vi "输入数据解析.vi"(0 "单个参数补充":dbl, 1 "从板号":dbl=1.0, 2 "主板二维码":string="BNET01", 3 "从板二维码":string="BNET01", 5 "主板引用":refnum<vi>, 7 "从板引用":refnum<vi>, 9 "主板选项":string="三级故障阀值", 11 "枚举":enum16{"主板", "从板"}(ring), 12 "快换":bool caption="快换写入") -> (4 "输出数组":dbl[][](array[numeric]), 6 "数组长度":dbl[](array[numeric]), 8 "循环次数":i32, 10 "命令":u32, 14 "名称":string[](array[string]), 15 "命令序号":u32[](array[numeric]))   [LabVIEW 2013] (continued)
          n307 = Build Array(u32 5 ("命令序号")) -> (w669:u32[])
          n308 = Insert Into Array(array=w655, index=w657, new element #1=w657, new element #2=1.0 ("新元素/子数组")) -> (w656:dbl[])
          n309 = Build Array(w656) -> (w664:dbl[][])
          n310 = Build Array("温度个数") -> (w660:string[])
        }
        frame "温度起始值" {
          n311 = Unbundle By Name(w709) -> ("项目信息"=w704:refnum<vi>)
          n312 = property class="Tbl (严格)"(reference=w704) -> ("Value"=w703:string[][])  [unwired: 1 in, 2 out]
          n313 = Index Array(array=w703, index (col)=1 ("禁用的索引 (列)")) -> (element=w705:string[])  [unwired: 1 in]
          n314 = Increment(x=w696) -> (x+1=w698:dbl)
          n315 = Multiply(x=w696, y=3.0) -> (x*y=w694:dbl)
          n316 = Add(x=w694, y=23.0) -> (x+y=w697:dbl)
          n317 = Array Subset(array=w705, index=w697, length=w698) -> (w707:string[])
          n318 = Fract/Exp String To Number(string=w707) -> (number=w692:dbl[])  [unwired: 4 out]
          n319 = for {
            tunnel: w692 -> [w716] mode=indexing
            shift-right: [w711] -> w691
            shift-left: dbl[] [] -> [w710]
            n320 = Quotient & Remainder(x=w716, y=256.0) -> (x-y*floor(x/y)=w713:dbl, floor(x/y)=w714:dbl)
            n321 = Build Array(w714, w713) -> (w712:dbl[])
            n322 = Insert Into Array(array=w710, new element=w712) -> (w711:dbl[])  [unwired: 1 in]
          }
          n323 = Build Array(62.0 ("元素")) -> (w702:dbl[])
          n324 = Build Array(u32 6 ("命令序号")) -> (w700:u32[])
          n325 = Build Array(w691) -> (w690:dbl[][])
          n326 = Build Array("温度起始值") -> (w686:string[])
        }
        frame "SOC" {
          # "SOC"
          n327 = Unbundle By Name(w737) -> ("一级故障 4"=w732:refnum<vi>)
          n328 = property class="Clust (严格)"(reference=w732) -> ("Value"=w731:T3)  [unwired: 1 in, 2 out]
          n329 = Unbundle By Name(w731) -> ("SOC(%)"=w729:dbl)
          n330 = call "输入分辨率计算-EV05.vi"("1字节?"=FALSE, "数值"=w729, "分辨率"=0.1) -> ("低字节"=w726:dbl, "高字节1"=w727:dbl)  [unwired: 2 in, 5 out]
          n331 = Build Array(w727, w726) -> (w738:dbl[])
          n332 = Two Button Dialog(message="输入SOC前请确认实际容量己输入" ("消息"), 1:"取消" ("F按钮名称（“取消”）"), 2:"确定" ("T按钮名称（“确定”）")) -> (T button?=w720:bool)
          n333 = case shown="假" w720 {
            tunnel: [0 1] -> w733
            frame False {
            }
            frame True {
            }
          }
          n334 = Build Array("SOC") -> (w721:string[])
          n335 = Build Array(w738) -> (w725:dbl[][])
          n336 = Build Array(2.0 ("单个参数补充")) -> (w724:dbl[])
          n337 = Build Array(u32 7 ("命令序号")) -> (w723:u32[])
        }
        frame "电池额定实际容量" {
          w754 = 256.0 ("y")
          w763 = 256.0 ("y")
          # "电池额定容量,实际容量"
          n338 = Unbundle By Name(w774) -> ("一级故障 4"=w761:refnum<vi>)
          n339 = property class="Clust (严格)"(reference=w761) -> ("Value"=w760:T3)  [unwired: 1 in, 2 out]
          n340 = Unbundle By Name(w760) -> ("电池额定容量(A)"=w758:dbl, "电池实际容量(A)"=w757:dbl)
          n341 = call "输入分辨率计算-EV05.vi"("1字节?"=TRUE, "数值 2"=w757, "数值"=w758, "分辨率"=0.001) -> ("高字节 2"=w750:dbl, "高字节1"=w756:dbl)  [unwired: 1 in, 5 out]
          n342 = Quotient & Remainder(x=w756, y=w763) -> (x-y*floor(x/y)=w767:dbl, floor(x/y)=w769:dbl)
          n343 = Quotient & Remainder(x=w750, y=w754) -> (x-y*floor(x/y)=w746:dbl, floor(x/y)=w751:dbl)
          n344 = Quotient & Remainder(x=w769, y=w763) -> (x-y*floor(x/y)=w766:dbl, floor(x/y)=w768:dbl)
          n345 = Quotient & Remainder(x=w751, y=w754) -> (x-y*floor(x/y)=w747:dbl, floor(x/y)=w752:dbl)
          n346 = Quotient & Remainder(x=w768, y=w763) -> (x-y*floor(x/y)=w765:dbl, floor(x/y)=w764:dbl)
          n347 = Quotient & Remainder(x=w752, y=w754) -> (x-y*floor(x/y)=w748:dbl, floor(x/y)=w753:dbl)
          n348 = Quotient & Remainder(x=w753, y=w754) -> (x-y*floor(x/y)=w749:dbl)  [unwired: 1 out]
          n349 = Quotient & Remainder(x=w764, y=w763) -> (x-y*floor(x/y)=w762:dbl)  [unwired: 1 out]
          n350 = Build Array(w762, w765, w766, w767, w749, w748, w747, w746) -> (w775:dbl[])
          n351 = Build Array(w775) -> (w745:dbl[][])
          n352 = Build Array(8.0 ("单个参数补充")) -> (w744:dbl[])
          n353 = Build Array(u32 8 ("命令序号")) -> (w743:u32[])
          n354 = Build Array("电池额定实际容量") -> (w741:string[])
        }
        frame "配置文件版本" {
          w787 = 8 ("长度")
          # "配置文件版本"
          n355 = Unbundle By Name(w789) -> ("一级故障 4"=w783:refnum<vi>)
          n356 = property class="Clust (严格)"(reference=w783) -> ("Value"=w782:T3)  [unwired: 1 in, 2 out]
          n357 = Unbundle By Name(w782) -> ("配置文件版本"=w781:string)
          n358 = String To Byte Array(string=w781) -> (unsigned byte array=w784:u8[])
          n359 = Array Subset(array=w784, length=w787) -> (w790:u8[])  [unwired: 1 in]
          n360 = Build Array(w790) -> (w780:u8[][])
          n361 = Build Array(w787) -> (w779:i32[])
          n362 = Build Array(u32 9 ("命令序号")) -> (w778:u32[])
          n363 = Build Array("配置文件版本") -> (w776:string[])
        }
        frame "参数修改记录" {
          n364 = Unbundle By Name(w813) -> ("一级故障 4"=w802:refnum<vi>)
          n365 = property class="Clust (严格)"(reference=w802) -> ("Value"=w801:T3)  [unwired: 1 in, 2 out]
          n366 = Unbundle By Name(w801) -> ("使用者"=w800:dbl)
          n367 = Quotient & Remainder(x=w800, y=256.0) -> (x-y*floor(x/y)=w797:dbl, floor(x/y)=w798:dbl)
          n368 = call "当前时间解析-8.6.vi"("需要秒？(T)"=TRUE) -> ("年"=w808:u8, "月"=w807:u8, "日"=w806:u8, "时"=w805:u8, "分"=w804:u8, "秒"=w803:u8)  [unwired: 13 out]
          n369 = Build Array(w798, w797, w808, w807, w806, w805, w804, w803) -> (w814:dbl[])
          n370 = Build Array(w814) -> (w796:dbl[][])
          n371 = Build Array(8.0 ("单个参数补充")) -> (w795:dbl[])
          n372 = Build Array(u32 10 ("命令序号")) -> (w794:u32[])
          n373 = Build Array("参数修改记录") -> (w791:string[])
        }
        frame "校正时钟" {
          n374 = call "当前时间解析-8.6.vi"("需要秒？(T)"=TRUE) -> ("年"=w826:u8, "月"=w825:u8, "日"=w824:u8, "时"=w823:u8, "分"=w822:u8, "秒"=w821:u8)  [unwired: 13 out]
          n375 = Build Array(w826, w825, w824, w823, w822, w821) -> (w831:u8[])
          n376 = Build Array(w831) -> (w820:u8[][])
          n377 = Build Array(6.0 ("单个参数补充")) -> (w819:dbl[])
          n378 = Build Array(u32 14 ("命令序号")) -> (w818:u32[])
          n379 = Build Array("校正时钟") -> (w815:string[])
        }
        frame "车牌号" {
          w843 = 8 ("长度")
          # "车牌号"
          n380 = Unbundle By Name(w845) -> ("一级故障 4"=w839:refnum<vi>)
          n381 = property class="Clust (严格)"(reference=w839) -> ("Value"=w838:T3)  [unwired: 1 in, 2 out]
          n382 = Unbundle By Name(w838) -> ("车架(牌)号"=w837:string)
          n383 = String To Byte Array(string=w837) -> (unsigned byte array=w840:u8[])
          n384 = Array Subset(array=w840, length=w843) -> (w846:u8[])  [unwired: 1 in]
          n385 = Build Array(w846) -> (w836:u8[][])
          n386 = Build Array(w843) -> (w835:i32[])
          n387 = Build Array("车牌号") -> (w832:string[])
          n388 = Build Array(u32 11 ("命令序号")) -> (w834:u32[])
        }
        frame "SOH" {
          n389 = Unbundle By Name(w863) -> ("一级故障 4"=w858:refnum<vi>)
          n390 = property class="Clust (严格)"(reference=w858) -> ("Value"=w857:T3)  [unwired: 1 in, 2 out]
          n391 = Unbundle By Name(w857) -> ("SOH(%)"=w856:dbl)
          n392 = call "输入分辨率计算-EV05.vi"("1字节?"=FALSE, "数值"=w856, "分辨率"=0.1) -> ("低字节"=w852:dbl, "高字节1"=w853:dbl)  [unwired: 2 in, 5 out]
          n393 = Build Array(w853, w852) -> (w864:dbl[])
          n394 = Build Array(w864) -> (w851:dbl[][])
          n395 = Build Array(2.0 ("单个参数补充")) -> (w850:dbl[])
          n396 = Build Array("SOH") -> (w847:string[])
          n397 = Build Array(u32 12 ("命令序号")) -> (w849:u32[])
        }
        frame "一级故障阀值" {
          n398 = Unbundle By Name(w870) -> ("一级故障"=w871:refnum<vi>)
          n399 = property class="Clust (严格)"(reference=w871) -> ("Value"=w869:T4)  [unwired: 1 in, 2 out]
          n400 = for {
            N: 17 -> [_]
            tunnel: w869 -> [w881]
            shift-right: [w878] -> w875
            shift-left: dbl[] [] -> [w879]
            i -> [w882]
            n401 = case shown="11" w882 {
              tunnel: w881 -> [w884 w891 w898 w905 w912 w918 w926 w934 w942 w950 w958 w966 w974 w982 w992 w999 w1003]
              tunnel: [w885 w892 w900 w907 w913 w921 w929 w937 w945 w953 w961 w967 w976 w984 w991 w998 w1005] -> w880
              frame 0, Default {
                # "总电压过高"
                n402 = Unbundle By Name(w884) -> ("总电压过高"=w883:dbl)
                n403 = call "输入分辨率计算-EV05.vi"("1字节?"=FALSE, "数值"=w883, "分辨率"=0.1) -> ("低字节"=w887:dbl, "高字节1"=w886:dbl)  [unwired: 2 in, 5 out]
                n404 = Build Array(w886, w887) -> (w885:dbl[])
              }
              frame 1 {
                # "总电压过低"
                n405 = Unbundle By Name(w891) -> ("总电压过低"=w890:dbl)
                n406 = call "输入分辨率计算-EV05.vi"("1字节?"=FALSE, "数值"=w890, "分辨率"=0.1) -> ("低字节"=w894:dbl, "高字节1"=w893:dbl)  [unwired: 2 in, 5 out]
                n407 = Build Array(w893, w894) -> (w892:dbl[])
              }
              frame 2 {
                # "温度过高"
                n408 = Unbundle By Name(w898) -> ("温度过高"=w897:dbl)
                n409 = call "输入分辨率计算-EV05.vi"("1字节?"=TRUE, "数值"=w897, "偏移量"=-40.0, "分辨率"=1.0) -> ("高字节1"=w901:dbl)  [unwired: 1 in, 6 out]
                n410 = Build Array(w901) -> (w900:dbl[])
              }
              frame 3 {
                # "温度过低"
                n411 = Unbundle By Name(w905) -> ("温度过低"=w904:dbl)
                n412 = call "输入分辨率计算-EV05.vi"("1字节?"=TRUE, "数值"=w904, "偏移量"=-40.0, "分辨率"=1.0) -> ("高字节1"=w908:dbl)  [unwired: 1 in, 6 out]
                n413 = Build Array(w908) -> (w907:dbl[])
              }
              frame 4 {
                # "整组温度不均衡"
                n414 = Unbundle By Name(w912) -> ("整组温度不均衡"=w911:dbl)
                n415 = call "输入分辨率计算-EV05.vi"("1字节?"=TRUE, "数值"=w911, "分辨率"=1.0) -> ("高字节1"=w914:dbl)  [unwired: 2 in, 6 out]
                n416 = Build Array(w914) -> (w913:dbl[])
              }
              frame 5 {
                # "单组电压不均衡"
                n417 = Unbundle By Name(w918) -> ("单组电压不均衡"=w917:dbl)
                n418 = call "输入分辨率计算-EV05.vi"("1字节?"=FALSE, "数值"=w917, "偏移量"=0.0, "分辨率"=0.001) -> ("低字节"=w919:dbl, "高字节1"=w922:dbl)  [unwired: 1 in, 5 out]
                n419 = Build Array(w922, w919) -> (w921:dbl[])
              }
              frame 6 {
                # "整组电压不均衡"
                n420 = Unbundle By Name(w926) -> ("整组电压不均衡"=w925:dbl)
                n421 = call "输入分辨率计算-EV05.vi"("1字节?"=FALSE, "数值"=w925, "偏移量"=0.0, "分辨率"=0.001) -> ("低字节"=w927:dbl, "高字节1"=w930:dbl)  [unwired: 1 in, 5 out]
                n422 = Build Array(w930, w927) -> (w929:dbl[])
              }
              frame 7 {
                # "单体电压过高"
                n423 = Unbundle By Name(w934) -> ("单体电压过高"=w933:dbl)
                n424 = call "输入分辨率计算-EV05.vi"("1字节?"=FALSE, "数值"=w933, "偏移量"=0.0, "分辨率"=0.001) -> ("低字节"=w935:dbl, "高字节1"=w938:dbl)  [unwired: 1 in, 5 out]
                n425 = Build Array(w938, w935) -> (w937:dbl[])
              }
              frame 8 {
                # "单体电压过低"
                n426 = Unbundle By Name(w942) -> ("单体电压过低"=w941:dbl)
                n427 = call "输入分辨率计算-EV05.vi"("1字节?"=FALSE, "数值"=w941, "偏移量"=0.0, "分辨率"=0.001) -> ("低字节"=w943:dbl, "高字节1"=w946:dbl)  [unwired: 1 in, 5 out]
                n428 = Build Array(w946, w943) -> (w945:dbl[])
              }
              frame 9 {
                # "充电电流过高"
                n429 = Unbundle By Name(w950) -> ("充电电流过高"=w949:dbl)
                n430 = call "输入分辨率计算-EV05.vi"("1字节?"=FALSE, "数值"=w949, "偏移量"=0.0, "分辨率"=0.1) -> ("低字节"=w951:dbl, "高字节1"=w954:dbl)  [unwired: 1 in, 5 out]
                n431 = Build Array(w954, w951) -> (w953:dbl[])
              }
              frame 10 {
                # "放电电流过高"
                n432 = Unbundle By Name(w958) -> ("放电电流过高"=w957:dbl)
                n433 = call "输入分辨率计算-EV05.vi"("1字节?"=FALSE, "数值"=w957, "偏移量"=0.0, "分辨率"=0.1) -> ("低字节"=w959:dbl, "高字节1"=w962:dbl)  [unwired: 1 in, 5 out]
                n434 = Build Array(w962, w959) -> (w961:dbl[])
              }
              frame 11 {
                # "单组温度不均衡"
                n435 = Unbundle By Name(w966) -> ("单组温度不均衡"=w965:dbl)
                n436 = call "输入分辨率计算-EV05.vi"("1字节?"=TRUE, "数值"=w965, "分辨率"=1.0) -> ("高字节1"=w968:dbl)  [unwired: 2 in, 6 out]
                n437 = Build Array(w968) -> (w967:dbl[])
              }
              frame 12 {
                # "SOC过高"
                n438 = Unbundle By Name(w974) -> ("SOC过高"=w973:dbl)
                n439 = call "输入分辨率计算-EV05.vi"("1字节?"=FALSE, "数值"=w973, "偏移量"=0.0, "分辨率"=0.1) -> ("低字节"=w971:dbl, "高字节1"=w972:dbl)  [unwired: 1 in, 5 out]
                n440 = Build Array(w972, w971) -> (w976:dbl[])
              }
              frame 13 {
                # "SOC过低"
                n441 = Unbundle By Name(w982) -> ("SOC过低"=w981:dbl)
                n442 = call "输入分辨率计算-EV05.vi"("1字节?"=FALSE, "数值"=w981, "偏移量"=0.0, "分辨率"=0.1) -> ("低字节"=w979:dbl, "高字节1"=w980:dbl)  [unwired: 1 in, 5 out]
                n443 = Build Array(w980, w979) -> (w984:dbl[])
              }
              frame 14 {
                # "内阻过大"
                n444 = Unbundle By Name(w992) -> ("内阻过大"=w990:dbl)
                n445 = call "输入分辨率计算-EV05.vi"("1字节?"=TRUE, "数值"=w990, "分辨率"=0.1) -> ("高字节1"=w987:dbl)  [unwired: 2 in, 6 out]
                n446 = Build Array(w987) -> (w991:dbl[])
              }
              frame 15 {
                # "极柱温度过高"
                n447 = Unbundle By Name(w999) -> ("极柱温度过高"=w997:dbl)
                n448 = call "输入分辨率计算-EV05.vi"("1字节?"=TRUE, "数值"=w997, "偏移量"=-40.0, "分辨率"=1.0) -> ("高字节1"=w994:dbl)  [unwired: 1 in, 6 out]
                n449 = Build Array(w994) -> (w998:dbl[])
              }
              frame 16 {
                # "SOH过低"
                n450 = Unbundle By Name(w1003) -> ("SOH过低"=w1002:dbl)
                n451 = call "输入分辨率计算-EV05.vi"("1字节?"=FALSE, "数值"=w1002, "偏移量"=0.0, "分辨率"=0.1) -> ("低字节"=w1001:dbl, "高字节1"=w1000:dbl)  [unwired: 1 in, 5 out]
                n452 = Build Array(w1000, w1001) -> (w1005:dbl[])
              }
            }
            n453 = Insert Into Array(array=w879, new element=w880) -> (w878:dbl[])  [unwired: 1 in]
          }
          n454 = Build Array(w875) -> (w874:dbl[][])
          n455 = Build Array("一级故障阀值") -> (w865:string[])
        }
        frame "温度过高" {
          n456 = Unbundle By Name(w1013) -> ("一级故障"=w1014:refnum<vi>)
          n457 = property class="Clust (严格)"(reference=w1014) -> ("Value"=w1012:T4)  [unwired: 1 in, 2 out]
          n458 = for {
            N: 17 -> [_]
            tunnel: w1012 -> [w1024]
            shift-right: [w1021] -> w1018
            shift-left: dbl[] [] -> [w1022]
            i -> [w1025]
            n459 = case shown="13" w1025 {
              tunnel: w1024 -> [w1026 w1037 w1048 w1058 w1068 w1078 w1090 w1102 w1114 w1126 w1138 w1150 w1164 w1186 w1198 w1207 w1216]
              tunnel: [w1027 w1038 w1049 w1059 w1069 w1080 w1092 w1104 w1116 w1128 w1140 w1151 w1173 w1189 w1197 w1206 w1218] -> w1023
              frame 0, Default {
                # "总电压过高"
                n460 = disable-structure shown="启用" {
                  disable-tunnel: [w1033 w1036] -> w1029
                  disable-tunnel: [w1032 w1036] -> w1028
                  disable-tunnel: w1026 -> [w1031 _]
                  frame Disabled {
                    n461 = Unbundle By Name(w1031) -> ("总电压过高"=w1030:dbl)
                    n462 = call "输入分辨率计算-EV05.vi"("1字节?"=FALSE, "数值"=w1030, "分辨率"=0.1) -> ("低字节"=w1033:dbl, "高字节1"=w1032:dbl)  [unwired: 2 in, 5 out]
                  }
                  frame Enabled {
                    w1036 = 255 ("高字节1")
                  }
                }
                n463 = Build Array(w1028, w1029) -> (w1027:i32[])
              }
              frame 1 {
                # "总电压过低"
                n464 = disable-structure shown="启用" {
                  disable-tunnel: [w1044 w1047] -> w1040
                  disable-tunnel: [w1043 w1047] -> w1039
                  disable-tunnel: w1037 -> [w1042 _]
                  frame Disabled {
                    n465 = Unbundle By Name(w1042) -> ("总电压过低"=w1041:dbl)
                    n466 = call "输入分辨率计算-EV05.vi"("1字节?"=FALSE, "数值"=w1041, "分辨率"=0.1) -> ("低字节"=w1044:dbl, "高字节1"=w1043:dbl)  [unwired: 2 in, 5 out]
                  }
                  frame Enabled {
                    w1047 = 255 ("高字节1")
                  }
                }
                n467 = Build Array(w1039, w1040) -> (w1038:i32[])
              }
              frame 2 {
                # "温度过高"
                n468 = disable-structure shown="启用" {
                  disable-tunnel: [w1054 255 ("高字节1")] -> w1050
                  disable-tunnel: w1048 -> [w1052 _]
                  frame Enabled {
                    n469 = Unbundle By Name(w1052) -> ("温度过高"=w1051:dbl)
                    n470 = call "输入分辨率计算-EV05.vi"("1字节?"=TRUE, "数值"=w1051, "偏移量"=-40.0, "分辨率"=1.0) -> ("高字节1"=w1054:dbl)  [unwired: 1 in, 6 out]
                  }
                  frame Disabled {
                  }
                }
                n471 = Build Array(w1050) -> (w1049:dbl[])
              }
              frame 3 {
                # "温度过低"
                n472 = disable-structure shown="启用" {
                  disable-tunnel: [w1064 255 ("高字节1")] -> w1060
                  disable-tunnel: w1058 -> [w1062 _]
                  frame Disabled {
                    n473 = Unbundle By Name(w1062) -> ("温度过低"=w1061:dbl)
                    n474 = call "输入分辨率计算-EV05.vi"("1字节?"=TRUE, "数值"=w1061, "偏移量"=-40.0, "分辨率"=1.0) -> ("高字节1"=w1064:dbl)  [unwired: 1 in, 6 out]
                  }
                  frame Enabled {
                  }
                }
                n475 = Build Array(w1060) -> (w1059:i32[])
              }
              frame 4 {
                # "整组温度不均衡"
                n476 = disable-structure shown="启用" {
                  disable-tunnel: [w1074 255 ("高字节1")] -> w1070
                  disable-tunnel: w1068 -> [w1072 _]
                  frame Disabled {
                    n477 = Unbundle By Name(w1072) -> ("整组温度不均衡"=w1071:dbl)
                    n478 = call "输入分辨率计算-EV05.vi"("1字节?"=TRUE, "数值"=w1071, "偏移量"=0.0, "分辨率"=1.0) -> ("高字节1"=w1074:dbl)  [unwired: 1 in, 6 out]
                  }
                  frame Enabled {
                  }
                }
                n479 = Build Array(w1070) -> (w1069:i32[])
              }
              frame 5 {
                # "单组电压不均衡"
                n480 = disable-structure shown="启用" {
                  disable-tunnel: [w1086 w1089] -> w1081
                  disable-tunnel: [w1084 w1089] -> w1079
                  disable-tunnel: w1078 -> [w1083 _]
                  frame Disabled {
                    n481 = Unbundle By Name(w1083) -> ("单组电压不均衡"=w1082:dbl)
                    n482 = call "输入分辨率计算-EV05.vi"("1字节?"=FALSE, "数值"=w1082, "偏移量"=0.0, "分辨率"=0.001) -> ("低字节"=w1084:dbl, "高字节1"=w1086:dbl)  [unwired: 1 in, 5 out]
                  }
                  frame Enabled {
                    w1089 = 255 ("高字节1")
                  }
                }
                n483 = Build Array(w1081, w1079) -> (w1080:i32[])
              }
              frame 6 {
                # "整组电压不均衡"
                n484 = disable-structure shown="启用" {
                  disable-tunnel: [w1098 w1101] -> w1093
                  disable-tunnel: [w1096 w1101] -> w1091
                  disable-tunnel: w1090 -> [w1095 _]
                  frame Disabled {
                    n485 = Unbundle By Name(w1095) -> ("整组电压不均衡"=w1094:dbl)
                    n486 = call "输入分辨率计算-EV05.vi"("1字节?"=FALSE, "数值"=w1094, "偏移量"=0.0, "分辨率"=0.001) -> ("低字节"=w1096:dbl, "高字节1"=w1098:dbl)  [unwired: 1 in, 5 out]
                  }
                  frame Enabled {
                    w1101 = 255 ("高字节1")
                  }
                }
                n487 = Build Array(w1093, w1091) -> (w1092:i32[])
              }
              frame 7 {
                # "单体电压过高"
                n488 = disable-structure shown="启用" {
                  disable-tunnel: [w1110 w1113] -> w1105
                  disable-tunnel: [w1108 w1113] -> w1103
                  disable-tunnel: w1102 -> [w1107 _]
                  frame Disabled {
                    n489 = Unbundle By Name(w1107) -> ("单体电压过高"=w1106:dbl)
                    n490 = call "输入分辨率计算-EV05.vi"("1字节?"=FALSE, "数值"=w1106, "偏移量"=0.0, "分辨率"=0.001) -> ("低字节"=w1108:dbl, "高字节1"=w1110:dbl)  [unwired: 1 in, 5 out]
                  }
                  frame Enabled {
                    w1113 = 255 ("高字节1")
                  }
                }
                n491 = Build Array(w1105, w1103) -> (w1104:i32[])
              }
              frame 8 {
                # "单体电压过低"
                n492 = disable-structure shown="启用" {
                  disable-tunnel: [w1122 w1125] -> w1117
                  disable-tunnel: [w1120 w1125] -> w1115
                  disable-tunnel: w1114 -> [w1119 _]
                  frame Disabled {
                    n493 = Unbundle By Name(w1119) -> ("单体电压过低"=w1118:dbl)
                    n494 = call "输入分辨率计算-EV05.vi"("1字节?"=FALSE, "数值"=w1118, "偏移量"=0.0, "分辨率"=0.001) -> ("低字节"=w1120:dbl, "高字节1"=w1122:dbl)  [unwired: 1 in, 5 out]
                  }
                  frame Enabled {
                    w1125 = 255 ("高字节1")
                  }
                }
                n495 = Build Array(w1117, w1115) -> (w1116:i32[])
              }
              frame 9 {
                # "充电电流过高"
                n496 = disable-structure shown="启用" {
                  disable-tunnel: [w1134 w1137] -> w1129
                  disable-tunnel: [w1132 w1137] -> w1127
                  disable-tunnel: w1126 -> [w1131 _]
                  frame Disabled {
                    n497 = Unbundle By Name(w1131) -> ("充电电流过高"=w1130:dbl)
                    n498 = call "输入分辨率计算-EV05.vi"("1字节?"=FALSE, "数值"=w1130, "偏移量"=-3000.0, "分辨率"=0.1) -> ("低字节"=w1132:dbl, "高字节1"=w1134:dbl)  [unwired: 1 in, 5 out]
                  }
                  frame Enabled {
                    w1137 = 255 ("高字节1")
                  }
                }
                n499 = Build Array(w1129, w1127) -> (w1128:i32[])
              }
              frame 10 {
                # "放电电流过高"
                n500 = disable-structure shown="启用" {
                  disable-tunnel: [w1146 w1149] -> w1141
                  disable-tunnel: [w1144 w1149] -> w1139
                  disable-tunnel: w1138 -> [w1143 _]
                  frame Disabled {
                    n501 = Unbundle By Name(w1143) -> ("放电电流过高"=w1142:dbl)
                    n502 = call "输入分辨率计算-EV05.vi"("1字节?"=FALSE, "数值"=w1142, "偏移量"=-3000.0, "分辨率"=0.1) -> ("低字节"=w1144:dbl, "高字节1"=w1146:dbl)  [unwired: 1 in, 5 out]
                  }
                  frame Enabled {
                    w1149 = 255 ("高字节1")
                  }
                }
                n503 = Build Array(w1141, w1139) -> (w1140:i32[])
              }
              frame 11 {
                # "单组温度不均衡"
                n504 = disable-structure shown="启用" {
                  disable-tunnel: [w1156 255 ("高字节1")] -> w1152
                  disable-tunnel: w1150 -> [w1154 _]
                  frame Disabled {
                    n505 = Unbundle By Name(w1154) -> ("单组温度不均衡"=w1153:dbl)
                    n506 = call "输入分辨率计算-EV05.vi"("1字节?"=TRUE, "数值"=w1153, "偏移量"=0.0, "分辨率"=1.0) -> ("高字节1"=w1156:dbl)  [unwired: 1 in, 6 out]
                  }
                  frame Enabled {
                  }
                }
                n507 = Build Array(w1152) -> (w1151:i32[])
              }
              frame 12 {
                # "SOC过高"
                n508 = Unbundle By Name(w1164) -> ("SOC过高"=w1163:dbl)
                n509 = call "输入分辨率计算-EV05.vi"("1字节?"=FALSE, "数值"=w1163, "偏移量"=0.0, "分辨率"=0.1) -> ("低字节"=w1165:dbl, "高字节1"=w1166:dbl)  [unwired: 1 in, 5 out]
                n510 = call "二进制解析-8.6.vi"("索引"=4, "数值"=w1166) -> ("低位子数组"=w1169:i32[])  [unwired: 3 out]
                n511 = call "二进制解析-8.6.vi"("索引"=4, "数值"=w1165) -> ("低位子数组"=w1161:i32[], "高位子数组"=w1168:i32[])  [unwired: 2 out]
                n512 = Insert Into Array(array=w1169, new element=w1168) -> (w1167:i32[])  [unwired: 1 in]
                n513 = call "数值二进制转十进制-8.6.vi"("子数组"=w1167) -> ("十进制数值"=w1162:i32)  [unwired: 4 out]
                n514 = disable-structure shown="启用" {
                  disable-tunnel: w1162 -> [w1177 _]
                  disable-tunnel: [w1177 255 ("高字节1")] -> w1160
                  disable-tunnel: [w1176 i32[] [] ("低位子数组 20")] -> _
                  disable-tunnel: w1161 -> [w1176 _]
                  frame Disabled {
                  }
                  frame Enabled {
                  }
                }
                n515 = Build Array(w1160, w1160) -> (w1173:i32[])
              }
              frame 13 {
                # "SOC过低"
                n516 = Unbundle By Name(w1186) -> ("SOC过低"=w1185:dbl)
                n517 = call "输入分辨率计算-EV05.vi"("1字节?"=FALSE, "数值"=w1185, "偏移量"=0.0, "分辨率"=0.1) -> ("低字节"=w1183:dbl, "高字节1"=w1184:dbl)  [unwired: 1 in, 5 out]
                n518 = call "二进制解析-8.6.vi"("索引"=4, "数值"=w1184) -> ("低位子数组"=w1181:i32[])  [unwired: 3 out]
                n519 = disable-structure shown="启用" {
                  disable-tunnel: w1183 -> [w1193 _]
                  disable-tunnel: [w1193 255 ("高字节1")] -> w1182
                  disable-tunnel: w1181 -> [w1192 _]
                  disable-tunnel: [_ 255 ("高字节1")] -> w1180
                  frame Disabled {
                    (unwired) i32[] [] ("低位子数组 4")
                  }
                  frame Enabled {
                  }
                }
                n520 = Build Array(w1180, w1182) -> (w1189:i32[])
              }
              frame 14 {
                # "内阻过大"
                n521 = disable-structure shown="启用" {
                  disable-tunnel: w1198 -> [w1203 _]
                  disable-tunnel: [w1199 255 ("高字节1")] -> w1196
                  frame Disabled {
                    n522 = Unbundle By Name(w1203) -> ("内阻过大"=w1202:dbl)
                    n523 = call "输入分辨率计算-EV05.vi"("1字节?"=TRUE, "数值"=w1202, "分辨率"=0.1) -> ("高字节1"=w1199:dbl)  [unwired: 2 in, 6 out]
                  }
                  frame Enabled {
                  }
                }
                n524 = Build Array(w1196) -> (w1197:i32[])
              }
              frame 15 {
                # "极柱温度过高"
                n525 = disable-structure shown="启用" {
                  disable-tunnel: w1207 -> [w1213 _]
                  disable-tunnel: [w1209 255 ("高字节1")] -> w1205
                  frame Disabled {
                    n526 = Unbundle By Name(w1213) -> ("极柱温度过高"=w1212:dbl)
                    n527 = call "输入分辨率计算-EV05.vi"("1字节?"=TRUE, "数值"=w1212, "偏移量"=-40.0, "分辨率"=1.0) -> ("高字节1"=w1209:dbl)  [unwired: 1 in, 6 out]
                  }
                  frame Enabled {
                  }
                }
                n528 = Build Array(w1205) -> (w1206:i32[])
              }
              frame 16 {
                # "SOH过低"
                n529 = disable-structure shown="启用" {
                  disable-tunnel: [w1230 w1238] -> w1217
                  disable-tunnel: w1216 -> [w1227 _]
                  disable-tunnel: [w1219 w1238] -> w1215
                  frame Disabled {
                    n530 = Unbundle By Name(w1227) -> ("SOH过低"=w1226:dbl)
                    n531 = call "输入分辨率计算-EV05.vi"("1字节?"=FALSE, "数值"=w1226, "偏移量"=0.0, "分辨率"=0.1) -> ("低字节"=w1228:dbl, "高字节1"=w1229:dbl)  [unwired: 1 in, 5 out]
                    n532 = call "二进制解析-8.6.vi"("索引"=4, "数值"=w1229) -> ("低位子数组"=w1232:i32[])  [unwired: 3 out]
                    n533 = call "二进制解析-8.6.vi"("索引"=4, "数值"=w1228) -> ("低位子数组"=w1221:i32[], "高位子数组"=w1231:i32[])  [unwired: 2 out]
                    n534 = call "二进制解析-8.6.vi"("索引"=4, "数值"=0) -> ("低位子数组"=w1222:i32[])  [unwired: 3 out]
                    n535 = Insert Into Array(array=w1232, new element=w1231) -> (w1225:i32[])  [unwired: 1 in]
                    n536 = Insert Into Array(array=w1221, new element=w1222) -> (w1220:i32[])  [unwired: 1 in]
                    n537 = call "数值二进制转十进制-8.6.vi"("子数组"=w1225) -> ("十进制数值"=w1230:i32)  [unwired: 4 out]
                    n538 = call "数值二进制转十进制-8.6.vi"("子数组"=w1220) -> ("十进制数值"=w1219:i32)  [unwired: 4 out]
                  }
                  frame Enabled {
                    w1238 = 255 ("高字节1")
                  }
                }
                n539 = Build Array(w1217, w1215) -> (w1218:i32[])
              }
            }
            n540 = Insert Into Array(array=w1022, new element=w1023) -> (w1021:dbl[])  [unwired: 1 in]
          }
          n541 = Build Array(w1018) -> (w1017:dbl[][])
          n542 = Build Array("一级故障阀值") -> (w1008:string[])
        }
        frame "总电压过高" {
          n543 = Unbundle By Name(w1244) -> ("一级故障"=w1245:refnum<vi>)
          n544 = property class="Clust (严格)"(reference=w1245) -> ("Value"=w1243:T4)  [unwired: 1 in, 2 out]
          n545 = for {
            N: 17 -> [_]
            tunnel: w1243 -> [w1255]
            shift-right: [w1252] -> w1249
            shift-left: dbl[] [] -> [w1253]
            i -> [w1256]
            n546 = case shown="13" w1256 {
              tunnel: w1255 -> [w1257 w1268 w1279 w1289 w1299 w1309 w1321 w1333 w1345 w1357 w1369 w1381 w1395 w1417 w1429 w1438 w1447]
              tunnel: [w1258 w1269 w1280 w1290 w1300 w1311 w1323 w1335 w1347 w1359 w1371 w1382 w1404 w1420 w1428 w1437 w1449] -> w1254
              frame 0, Default {
                # "总电压过高"
                n547 = disable-structure shown="启用" {
                  disable-tunnel: [w1264 w1267] -> w1260
                  disable-tunnel: [w1263 w1267] -> w1259
                  disable-tunnel: w1257 -> [w1262 _]
                  frame Enabled {
                    n548 = Unbundle By Name(w1262) -> ("总电压过高"=w1261:dbl)
                    n549 = call "输入分辨率计算-EV05.vi"("1字节?"=FALSE, "数值"=w1261, "分辨率"=0.1) -> ("低字节"=w1264:dbl, "高字节1"=w1263:dbl)  [unwired: 2 in, 5 out]
                  }
                  frame Disabled {
                    w1267 = 255 ("高字节1")
                  }
                }
                n550 = Build Array(w1259, w1260) -> (w1258:dbl[])
              }
              frame 1 {
                # "总电压过低"
                n551 = disable-structure shown="启用" {
                  disable-tunnel: [w1275 w1278] -> w1271
                  disable-tunnel: [w1274 w1278] -> w1270
                  disable-tunnel: w1268 -> [w1273 _]
                  frame Disabled {
                    n552 = Unbundle By Name(w1273) -> ("总电压过低"=w1272:dbl)
                    n553 = call "输入分辨率计算-EV05.vi"("1字节?"=FALSE, "数值"=w1272, "分辨率"=0.1) -> ("低字节"=w1275:dbl, "高字节1"=w1274:dbl)  [unwired: 2 in, 5 out]
                  }
                  frame Enabled {
                    w1278 = 255 ("高字节1")
                  }
                }
                n554 = Build Array(w1270, w1271) -> (w1269:i32[])
              }
              frame 2 {
                # "温度过高"
                n555 = disable-structure shown="启用" {
                  disable-tunnel: [w1285 255 ("高字节1")] -> w1281
                  disable-tunnel: w1279 -> [w1283 _]
                  frame Disabled {
                    n556 = Unbundle By Name(w1283) -> ("温度过高"=w1282:dbl)
                    n557 = call "输入分辨率计算-EV05.vi"("1字节?"=TRUE, "数值"=w1282, "偏移量"=-40.0, "分辨率"=1.0) -> ("高字节1"=w1285:dbl)  [unwired: 1 in, 6 out]
                  }
                  frame Enabled {
                  }
                }
                n558 = Build Array(w1281) -> (w1280:i32[])
              }
              frame 3 {
                # "温度过低"
                n559 = disable-structure shown="启用" {
                  disable-tunnel: [w1295 255 ("高字节1")] -> w1291
                  disable-tunnel: w1289 -> [w1293 _]
                  frame Disabled {
                    n560 = Unbundle By Name(w1293) -> ("温度过低"=w1292:dbl)
                    n561 = call "输入分辨率计算-EV05.vi"("1字节?"=TRUE, "数值"=w1292, "偏移量"=-40.0, "分辨率"=1.0) -> ("高字节1"=w1295:dbl)  [unwired: 1 in, 6 out]
                  }
                  frame Enabled {
                  }
                }
                n562 = Build Array(w1291) -> (w1290:i32[])
              }
              frame 4 {
                # "整组温度不均衡"
                n563 = disable-structure shown="启用" {
                  disable-tunnel: [w1305 255 ("高字节1")] -> w1301
                  disable-tunnel: w1299 -> [w1303 _]
                  frame Disabled {
                    n564 = Unbundle By Name(w1303) -> ("整组温度不均衡"=w1302:dbl)
                    n565 = call "输入分辨率计算-EV05.vi"("1字节?"=TRUE, "数值"=w1302, "偏移量"=0.0, "分辨率"=1.0) -> ("高字节1"=w1305:dbl)  [unwired: 1 in, 6 out]
                  }
                  frame Enabled {
                  }
                }
                n566 = Build Array(w1301) -> (w1300:i32[])
              }
              frame 5 {
                # "单组电压不均衡"
                n567 = disable-structure shown="启用" {
                  disable-tunnel: [w1317 w1320] -> w1312
                  disable-tunnel: [w1315 w1320] -> w1310
                  disable-tunnel: w1309 -> [w1314 _]
                  frame Disabled {
                    n568 = Unbundle By Name(w1314) -> ("单组电压不均衡"=w1313:dbl)
                    n569 = call "输入分辨率计算-EV05.vi"("1字节?"=FALSE, "数值"=w1313, "偏移量"=0.0, "分辨率"=0.001) -> ("低字节"=w1315:dbl, "高字节1"=w1317:dbl)  [unwired: 1 in, 5 out]
                  }
                  frame Enabled {
                    w1320 = 255 ("高字节1")
                  }
                }
                n570 = Build Array(w1312, w1310) -> (w1311:i32[])
              }
              frame 6 {
                # "整组电压不均衡"
                n571 = disable-structure shown="启用" {
                  disable-tunnel: [w1329 w1332] -> w1324
                  disable-tunnel: [w1327 w1332] -> w1322
                  disable-tunnel: w1321 -> [w1326 _]
                  frame Disabled {
                    n572 = Unbundle By Name(w1326) -> ("整组电压不均衡"=w1325:dbl)
                    n573 = call "输入分辨率计算-EV05.vi"("1字节?"=FALSE, "数值"=w1325, "偏移量"=0.0, "分辨率"=0.001) -> ("低字节"=w1327:dbl, "高字节1"=w1329:dbl)  [unwired: 1 in, 5 out]
                  }
                  frame Enabled {
                    w1332 = 255 ("高字节1")
                  }
                }
                n574 = Build Array(w1324, w1322) -> (w1323:i32[])
              }
              frame 7 {
                # "单体电压过高"
                n575 = disable-structure shown="启用" {
                  disable-tunnel: [w1341 w1344] -> w1336
                  disable-tunnel: [w1339 w1344] -> w1334
                  disable-tunnel: w1333 -> [w1338 _]
                  frame Disabled {
                    n576 = Unbundle By Name(w1338) -> ("单体电压过高"=w1337:dbl)
                    n577 = call "输入分辨率计算-EV05.vi"("1字节?"=FALSE, "数值"=w1337, "偏移量"=0.0, "分辨率"=0.001) -> ("低字节"=w1339:dbl, "高字节1"=w1341:dbl)  [unwired: 1 in, 5 out]
                  }
                  frame Enabled {
                    w1344 = 255 ("高字节1")
                  }
                }
                n578 = Build Array(w1336, w1334) -> (w1335:i32[])
              }
              frame 8 {
                # "单体电压过低"
                n579 = disable-structure shown="启用" {
                  disable-tunnel: [w1353 w1356] -> w1348
                  disable-tunnel: [w1351 w1356] -> w1346
                  disable-tunnel: w1345 -> [w1350 _]
                  frame Disabled {
                    n580 = Unbundle By Name(w1350) -> ("单体电压过低"=w1349:dbl)
                    n581 = call "输入分辨率计算-EV05.vi"("1字节?"=FALSE, "数值"=w1349, "偏移量"=0.0, "分辨率"=0.001) -> ("低字节"=w1351:dbl, "高字节1"=w1353:dbl)  [unwired: 1 in, 5 out]
                  }
                  frame Enabled {
                    w1356 = 255 ("高字节1")
                  }
                }
                n582 = Build Array(w1348, w1346) -> (w1347:i32[])
              }
              frame 9 {
                # "充电电流过高"
                n583 = disable-structure shown="启用" {
                  disable-tunnel: [w1365 w1368] -> w1360
                  disable-tunnel: [w1363 w1368] -> w1358
                  disable-tunnel: w1357 -> [w1362 _]
                  frame Disabled {
                    n584 = Unbundle By Name(w1362) -> ("充电电流过高"=w1361:dbl)
                    n585 = call "输入分辨率计算-EV05.vi"("1字节?"=FALSE, "数值"=w1361, "偏移量"=-3000.0, "分辨率"=0.1) -> ("低字节"=w1363:dbl, "高字节1"=w1365:dbl)  [unwired: 1 in, 5 out]
                  }
                  frame Enabled {
                    w1368 = 255 ("高字节1")
                  }
                }
                n586 = Build Array(w1360, w1358) -> (w1359:i32[])
              }
              frame 10 {
                # "放电电流过高"
                n587 = disable-structure shown="启用" {
                  disable-tunnel: [w1377 w1380] -> w1372
                  disable-tunnel: [w1375 w1380] -> w1370
                  disable-tunnel: w1369 -> [w1374 _]
                  frame Disabled {
                    n588 = Unbundle By Name(w1374) -> ("放电电流过高"=w1373:dbl)
                    n589 = call "输入分辨率计算-EV05.vi"("1字节?"=FALSE, "数值"=w1373, "偏移量"=-3000.0, "分辨率"=0.1) -> ("低字节"=w1375:dbl, "高字节1"=w1377:dbl)  [unwired: 1 in, 5 out]
                  }
                  frame Enabled {
                    w1380 = 255 ("高字节1")
                  }
                }
                n590 = Build Array(w1372, w1370) -> (w1371:i32[])
              }
              frame 11 {
                # "单组温度不均衡"
                n591 = disable-structure shown="启用" {
                  disable-tunnel: [w1387 255 ("高字节1")] -> w1383
                  disable-tunnel: w1381 -> [w1385 _]
                  frame Disabled {
                    n592 = Unbundle By Name(w1385) -> ("单组温度不均衡"=w1384:dbl)
                    n593 = call "输入分辨率计算-EV05.vi"("1字节?"=TRUE, "数值"=w1384, "偏移量"=0.0, "分辨率"=1.0) -> ("高字节1"=w1387:dbl)  [unwired: 1 in, 6 out]
                  }
                  frame Enabled {
                  }
                }
                n594 = Build Array(w1383) -> (w1382:i32[])
              }
              frame 12 {
                # "SOC过高"
                n595 = Unbundle By Name(w1395) -> ("SOC过高"=w1394:dbl)
                n596 = call "输入分辨率计算-EV05.vi"("1字节?"=FALSE, "数值"=w1394, "偏移量"=0.0, "分辨率"=0.1) -> ("低字节"=w1396:dbl, "高字节1"=w1397:dbl)  [unwired: 1 in, 5 out]
                n597 = call "二进制解析-8.6.vi"("索引"=4, "数值"=w1397) -> ("低位子数组"=w1400:i32[])  [unwired: 3 out]
                n598 = call "二进制解析-8.6.vi"("索引"=4, "数值"=w1396) -> ("低位子数组"=w1392:i32[], "高位子数组"=w1399:i32[])  [unwired: 2 out]
                n599 = Insert Into Array(array=w1400, new element=w1399) -> (w1398:i32[])  [unwired: 1 in]
                n600 = call "数值二进制转十进制-8.6.vi"("子数组"=w1398) -> ("十进制数值"=w1393:i32)  [unwired: 4 out]
                n601 = disable-structure shown="启用" {
                  disable-tunnel: w1393 -> [w1408 _]
                  disable-tunnel: [w1408 255 ("高字节1")] -> w1391
                  disable-tunnel: [w1407 i32[] [] ("低位子数组 20")] -> _
                  disable-tunnel: w1392 -> [w1407 _]
                  frame Disabled {
                  }
                  frame Enabled {
                  }
                }
                n602 = Build Array(w1391, w1391) -> (w1404:i32[])
              }
              frame 13 {
                # "SOC过低"
                n603 = Unbundle By Name(w1417) -> ("SOC过低"=w1416:dbl)
                n604 = call "输入分辨率计算-EV05.vi"("1字节?"=FALSE, "数值"=w1416, "偏移量"=0.0, "分辨率"=0.1) -> ("低字节"=w1414:dbl, "高字节1"=w1415:dbl)  [unwired: 1 in, 5 out]
                n605 = call "二进制解析-8.6.vi"("索引"=4, "数值"=w1415) -> ("低位子数组"=w1412:i32[])  [unwired: 3 out]
                n606 = disable-structure shown="启用" {
                  disable-tunnel: w1414 -> [w1424 _]
                  disable-tunnel: [w1424 255 ("高字节1")] -> w1413
                  disable-tunnel: w1412 -> [w1423 _]
                  disable-tunnel: [_ 255 ("高字节1")] -> w1411
                  frame Disabled {
                    (unwired) i32[] [] ("低位子数组 4")
                  }
                  frame Enabled {
                  }
                }
                n607 = Build Array(w1411, w1413) -> (w1420:i32[])
              }
              frame 14 {
                # "内阻过大"
                n608 = disable-structure shown="启用" {
                  disable-tunnel: w1429 -> [w1434 _]
                  disable-tunnel: [w1430 255 ("高字节1")] -> w1427
                  frame Disabled {
                    n609 = Unbundle By Name(w1434) -> ("内阻过大"=w1433:dbl)
                    n610 = call "输入分辨率计算-EV05.vi"("1字节?"=TRUE, "数值"=w1433, "分辨率"=0.1) -> ("高字节1"=w1430:dbl)  [unwired: 2 in, 6 out]
                  }
                  frame Enabled {
                  }
                }
                n611 = Build Array(w1427) -> (w1428:i32[])
              }
              frame 15 {
                # "极柱温度过高"
                n612 = disable-structure shown="启用" {
                  disable-tunnel: w1438 -> [w1444 _]
                  disable-tunnel: [w1440 255 ("高字节1")] -> w1436
                  frame Disabled {
                    n613 = Unbundle By Name(w1444) -> ("极柱温度过高"=w1443:dbl)
                    n614 = call "输入分辨率计算-EV05.vi"("1字节?"=TRUE, "数值"=w1443, "偏移量"=-40.0, "分辨率"=1.0) -> ("高字节1"=w1440:dbl)  [unwired: 1 in, 6 out]
                  }
                  frame Enabled {
                  }
                }
                n615 = Build Array(w1436) -> (w1437:i32[])
              }
              frame 16 {
                # "SOH过低"
                n616 = disable-structure shown="启用" {
                  disable-tunnel: [w1461 w1469] -> w1448
                  disable-tunnel: w1447 -> [w1458 _]
                  disable-tunnel: [w1450 w1469] -> w1446
                  frame Disabled {
                    n617 = Unbundle By Name(w1458) -> ("SOH过低"=w1457:dbl)
                    n618 = call "输入分辨率计算-EV05.vi"("1字节?"=FALSE, "数值"=w1457, "偏移量"=0.0, "分辨率"=0.1) -> ("低字节"=w1459:dbl, "高字节1"=w1460:dbl)  [unwired: 1 in, 5 out]
                    n619 = call "二进制解析-8.6.vi"("索引"=4, "数值"=w1460) -> ("低位子数组"=w1463:i32[])  [unwired: 3 out]
                    n620 = call "二进制解析-8.6.vi"("索引"=4, "数值"=w1459) -> ("低位子数组"=w1452:i32[], "高位子数组"=w1462:i32[])  [unwired: 2 out]
                    n621 = call "二进制解析-8.6.vi"("索引"=4, "数值"=0) -> ("低位子数组"=w1453:i32[])  [unwired: 3 out]
                    n622 = Insert Into Array(array=w1463, new element=w1462) -> (w1456:i32[])  [unwired: 1 in]
                    n623 = Insert Into Array(array=w1452, new element=w1453) -> (w1451:i32[])  [unwired: 1 in]
                    n624 = call "数值二进制转十进制-8.6.vi"("子数组"=w1456) -> ("十进制数值"=w1461:i32)  [unwired: 4 out]
                    n625 = call "数值二进制转十进制-8.6.vi"("子数组"=w1451) -> ("十进制数值"=w1450:i32)  [unwired: 4 out]
                  }
                  frame Enabled {
                    w1469 = 255 ("高字节1")
                  }
                }
                n626 = Build Array(w1448, w1446) -> (w1449:i32[])
              }
            }
            n627 = Insert Into Array(array=w1253, new element=w1254) -> (w1252:dbl[])  [unwired: 1 in]
          }
          n628 = Build Array(w1249) -> (w1248:dbl[][])
          n629 = Build Array("一级故障阀值") -> (w1239:string[])
        }
        frame "总电压过低" {
          n630 = Unbundle By Name(w1475) -> ("一级故障"=w1476:refnum<vi>)
          n631 = property class="Clust (严格)"(reference=w1476) -> ("Value"=w1474:T4)  [unwired: 1 in, 2 out]
          n632 = for {
            N: 17 -> [_]
            tunnel: w1474 -> [w1486]
            shift-right: [w1483] -> w1480
            shift-left: dbl[] [] -> [w1484]
            i -> [w1487]
            n633 = case shown="13" w1487 {
              tunnel: w1486 -> [w1488 w1499 w1510 w1520 w1530 w1540 w1552 w1564 w1576 w1588 w1600 w1612 w1626 w1648 w1660 w1669 w1678]
              tunnel: [w1489 w1500 w1511 w1521 w1531 w1542 w1554 w1566 w1578 w1590 w1602 w1613 w1635 w1651 w1659 w1668 w1680] -> w1485
              frame 0, Default {
                # "总电压过高"
                n634 = disable-structure shown="启用" {
                  disable-tunnel: [w1495 w1498] -> w1491
                  disable-tunnel: [w1494 w1498] -> w1490
                  disable-tunnel: w1488 -> [w1493 _]
                  frame Disabled {
                    n635 = Unbundle By Name(w1493) -> ("总电压过高"=w1492:dbl)
                    n636 = call "输入分辨率计算-EV05.vi"("1字节?"=FALSE, "数值"=w1492, "分辨率"=0.1) -> ("低字节"=w1495:dbl, "高字节1"=w1494:dbl)  [unwired: 2 in, 5 out]
                  }
                  frame Enabled {
                    w1498 = 255 ("高字节1")
                  }
                }
                n637 = Build Array(w1490, w1491) -> (w1489:i32[])
              }
              frame 1 {
                # "总电压过低"
                n638 = disable-structure shown="启用" {
                  disable-tunnel: [w1506 w1509] -> w1502
                  disable-tunnel: [w1505 w1509] -> w1501
                  disable-tunnel: w1499 -> [w1504 _]
                  frame Enabled {
                    n639 = Unbundle By Name(w1504) -> ("总电压过低"=w1503:dbl)
                    n640 = call "输入分辨率计算-EV05.vi"("1字节?"=FALSE, "数值"=w1503, "分辨率"=0.1) -> ("低字节"=w1506:dbl, "高字节1"=w1505:dbl)  [unwired: 2 in, 5 out]
                  }
                  frame Disabled {
                    w1509 = 255 ("高字节1")
                  }
                }
                n641 = Build Array(w1501, w1502) -> (w1500:dbl[])
              }
              frame 2 {
                # "温度过高"
                n642 = disable-structure shown="启用" {
                  disable-tunnel: [w1516 255 ("高字节1")] -> w1512
                  disable-tunnel: w1510 -> [w1514 _]
                  frame Disabled {
                    n643 = Unbundle By Name(w1514) -> ("温度过高"=w1513:dbl)
                    n644 = call "输入分辨率计算-EV05.vi"("1字节?"=TRUE, "数值"=w1513, "偏移量"=-40.0, "分辨率"=1.0) -> ("高字节1"=w1516:dbl)  [unwired: 1 in, 6 out]
                  }
                  frame Enabled {
                  }
                }
                n645 = Build Array(w1512) -> (w1511:i32[])
              }
              frame 3 {
                # "温度过低"
                n646 = disable-structure shown="启用" {
                  disable-tunnel: [w1526 255 ("高字节1")] -> w1522
                  disable-tunnel: w1520 -> [w1524 _]
                  frame Disabled {
                    n647 = Unbundle By Name(w1524) -> ("温度过低"=w1523:dbl)
                    n648 = call "输入分辨率计算-EV05.vi"("1字节?"=TRUE, "数值"=w1523, "偏移量"=-40.0, "分辨率"=1.0) -> ("高字节1"=w1526:dbl)  [unwired: 1 in, 6 out]
                  }
                  frame Enabled {
                  }
                }
                n649 = Build Array(w1522) -> (w1521:i32[])
              }
              frame 4 {
                # "整组温度不均衡"
                n650 = disable-structure shown="启用" {
                  disable-tunnel: [w1536 255 ("高字节1")] -> w1532
                  disable-tunnel: w1530 -> [w1534 _]
                  frame Disabled {
                    n651 = Unbundle By Name(w1534) -> ("整组温度不均衡"=w1533:dbl)
                    n652 = call "输入分辨率计算-EV05.vi"("1字节?"=TRUE, "数值"=w1533, "偏移量"=0.0, "分辨率"=1.0) -> ("高字节1"=w1536:dbl)  [unwired: 1 in, 6 out]
                  }
                  frame Enabled {
                  }
                }
                n653 = Build Array(w1532) -> (w1531:i32[])
              }
              frame 5 {
                # "单组电压不均衡"
                n654 = disable-structure shown="启用" {
                  disable-tunnel: [w1548 w1551] -> w1543
                  disable-tunnel: [w1546 w1551] -> w1541
                  disable-tunnel: w1540 -> [w1545 _]
                  frame Disabled {
                    n655 = Unbundle By Name(w1545) -> ("单组电压不均衡"=w1544:dbl)
                    n656 = call "输入分辨率计算-EV05.vi"("1字节?"=FALSE, "数值"=w1544, "偏移量"=0.0, "分辨率"=0.001) -> ("低字节"=w1546:dbl, "高字节1"=w1548:dbl)  [unwired: 1 in, 5 out]
                  }
                  frame Enabled {
                    w1551 = 255 ("高字节1")
                  }
                }
                n657 = Build Array(w1543, w1541) -> (w1542:i32[])
              }
              frame 6 {
                # "整组电压不均衡"
                n658 = disable-structure shown="启用" {
                  disable-tunnel: [w1560 w1563] -> w1555
                  disable-tunnel: [w1558 w1563] -> w1553
                  disable-tunnel: w1552 -> [w1557 _]
                  frame Disabled {
                    n659 = Unbundle By Name(w1557) -> ("整组电压不均衡"=w1556:dbl)
                    n660 = call "输入分辨率计算-EV05.vi"("1字节?"=FALSE, "数值"=w1556, "偏移量"=0.0, "分辨率"=0.001) -> ("低字节"=w1558:dbl, "高字节1"=w1560:dbl)  [unwired: 1 in, 5 out]
                  }
                  frame Enabled {
                    w1563 = 255 ("高字节1")
                  }
                }
                n661 = Build Array(w1555, w1553) -> (w1554:i32[])
              }
              frame 7 {
                # "单体电压过高"
                n662 = disable-structure shown="启用" {
                  disable-tunnel: [w1572 w1575] -> w1567
                  disable-tunnel: [w1570 w1575] -> w1565
                  disable-tunnel: w1564 -> [w1569 _]
                  frame Disabled {
                    n663 = Unbundle By Name(w1569) -> ("单体电压过高"=w1568:dbl)
                    n664 = call "输入分辨率计算-EV05.vi"("1字节?"=FALSE, "数值"=w1568, "偏移量"=0.0, "分辨率"=0.001) -> ("低字节"=w1570:dbl, "高字节1"=w1572:dbl)  [unwired: 1 in, 5 out]
                  }
                  frame Enabled {
                    w1575 = 255 ("高字节1")
                  }
                }
                n665 = Build Array(w1567, w1565) -> (w1566:i32[])
              }
              frame 8 {
                # "单体电压过低"
                n666 = disable-structure shown="启用" {
                  disable-tunnel: [w1584 w1587] -> w1579
                  disable-tunnel: [w1582 w1587] -> w1577
                  disable-tunnel: w1576 -> [w1581 _]
                  frame Disabled {
                    n667 = Unbundle By Name(w1581) -> ("单体电压过低"=w1580:dbl)
                    n668 = call "输入分辨率计算-EV05.vi"("1字节?"=FALSE, "数值"=w1580, "偏移量"=0.0, "分辨率"=0.001) -> ("低字节"=w1582:dbl, "高字节1"=w1584:dbl)  [unwired: 1 in, 5 out]
                  }
                  frame Enabled {
                    w1587 = 255 ("高字节1")
                  }
                }
                n669 = Build Array(w1579, w1577) -> (w1578:i32[])
              }
              frame 9 {
                # "充电电流过高"
                n670 = disable-structure shown="启用" {
                  disable-tunnel: [w1596 w1599] -> w1591
                  disable-tunnel: [w1594 w1599] -> w1589
                  disable-tunnel: w1588 -> [w1593 _]
                  frame Disabled {
                    n671 = Unbundle By Name(w1593) -> ("充电电流过高"=w1592:dbl)
                    n672 = call "输入分辨率计算-EV05.vi"("1字节?"=FALSE, "数值"=w1592, "偏移量"=-3000.0, "分辨率"=0.1) -> ("低字节"=w1594:dbl, "高字节1"=w1596:dbl)  [unwired: 1 in, 5 out]
                  }
                  frame Enabled {
                    w1599 = 255 ("高字节1")
                  }
                }
                n673 = Build Array(w1591, w1589) -> (w1590:i32[])
              }
              frame 10 {
                # "放电电流过高"
                n674 = disable-structure shown="启用" {
                  disable-tunnel: [w1608 w1611] -> w1603
                  disable-tunnel: [w1606 w1611] -> w1601
                  disable-tunnel: w1600 -> [w1605 _]
                  frame Disabled {
                    n675 = Unbundle By Name(w1605) -> ("放电电流过高"=w1604:dbl)
                    n676 = call "输入分辨率计算-EV05.vi"("1字节?"=FALSE, "数值"=w1604, "偏移量"=-3000.0, "分辨率"=0.1) -> ("低字节"=w1606:dbl, "高字节1"=w1608:dbl)  [unwired: 1 in, 5 out]
                  }
                  frame Enabled {
                    w1611 = 255 ("高字节1")
                  }
                }
                n677 = Build Array(w1603, w1601) -> (w1602:i32[])
              }
              frame 11 {
                # "单组温度不均衡"
                n678 = disable-structure shown="启用" {
                  disable-tunnel: [w1618 255 ("高字节1")] -> w1614
                  disable-tunnel: w1612 -> [w1616 _]
                  frame Disabled {
                    n679 = Unbundle By Name(w1616) -> ("单组温度不均衡"=w1615:dbl)
                    n680 = call "输入分辨率计算-EV05.vi"("1字节?"=TRUE, "数值"=w1615, "偏移量"=0.0, "分辨率"=1.0) -> ("高字节1"=w1618:dbl)  [unwired: 1 in, 6 out]
                  }
                  frame Enabled {
                  }
                }
